vi "status_read.vi"(7 "references":T1, 8 "error in (no error)":errorcluster) -> (0 "error out":errorcluster, 3 "status":T3 {"auto_elapsed_time" format="%<%H:%M:%S%2u>t"})   [LabVIEW 2015, in "lv-recipe-machine.lvlib"]
doc: "This VI can be used to read the current status from the module (public). If you want to ensure that you're getting recently updated data rather than the most recent data, you can include a value for timeout. It's default is 0, in the case the default is used, it returns the most recent value (even if it's never been updated). If the timeout is non-zero and there's no new value, it will output a module specific error noting that the status notifier has timed out."
uses:
  lv-recipe-machine.lvlib
  _controls/status.ctl
  _controls/mode.ctl
  _controls/manual_state.ctl
  _controls/automatic_state.ctl
  _controls/references.ctl
  _controls/input.ctl
  _controls/input_command.ctl
  _controls/output.ctl
  _controls/data.ctl
  _controls/configuration.ctl
  _controls/recipe_data.ctl
  _controls/recipe_step.ctl
  <userlib>/antonio-alexander/lv-waitgroup/public/_controls/api_waitgroup.ctl
  _controls/change.ctl
  <userlib>/antonio-alexander/lv-waitgroup/lv-waitgroup.lvlib
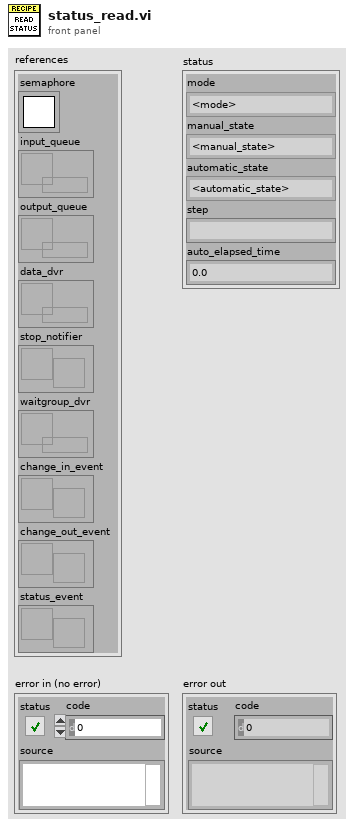
[diagram p1: front panel]
types:
  T1 = typedef "lv-recipe-machine.lvlib/references.ctl" = cluster{"semaphore":T2, "input_queue":refnum<queue>, "output_queue":refnum<queue>, "data_dvr":refnum<data-value>, "stop_notifier":refnum<notifier>, "waitgroup_dvr":refnum<data-value>, "change_in_event":refnum<user-event>, "change_out_event":refnum<user-event>, "status_event":refnum<user-event>}
  T2 = typedef "Semaphore RefNum" = refnum<k1>
  T3 = typedef "lv-recipe-machine.lvlib/status.ctl" = cluster{"mode":T4, "manual_state":T5, "automatic_state":T6, "step":string, "auto_elapsed_time":dbl}
  T4 = typedef "lv-recipe-machine.lvlib/mode.ctl" = enum16{"<mode>", "manual", "automatic", "<null>"}
  T5 = typedef "lv-recipe-machine.lvlib/manual_state.ctl" = enum16{"<manual_state>", "failed", "action", "running", "idle", "<null>"}
  T6 = typedef "lv-recipe-machine.lvlib/automatic_state.ctl" = enum16{"<automatic_state>", "failed", "idle", "running", "paused", "transition", "stopped", "<null>"}
  T7 = typedef "lv-recipe-machine.lvlib/data.ctl" = cluster{"configuration":T8, "working":cluster{"recipe_data":T9, "api_waitgroup":T11}}
  T8 = typedef "lv-recipe-machine.lvlib/configuration.ctl" = cluster{"max_processes":i32}
  T9 = typedef "lv-recipe-machine.lvlib/recipe_data.ctl" = cluster{"mode":T4, "manual_state":T5, "automatic_state":T6, "previous_automatic_state":T6, "error":errorcluster, "manual":cluster{"step_action":string, "data":variant, "actions":variant}, "automatic":cluster{"data":variant, "steps":variant, "criteria":variant, "transition":string, "index":i32, "recipe []":T10[]}}
  T10 = typedef "lv-recipe-machine.lvlib/recipe_step.ctl" = cluster{"step":string, "data":variant}
  T11 = typedef "lv-waitgroup.lvlib/api_waitgroup.ctl" = cluster{"waitgroups":refnum<data-value>, "waitgroup":string}
  T12 = cluster{"step_action":string, "data":variant, "actions":variant}
  T13 = cluster{"data":variant, "steps":variant, "criteria":variant, "transition":string, "index":i32, "recipe []":T10[]}
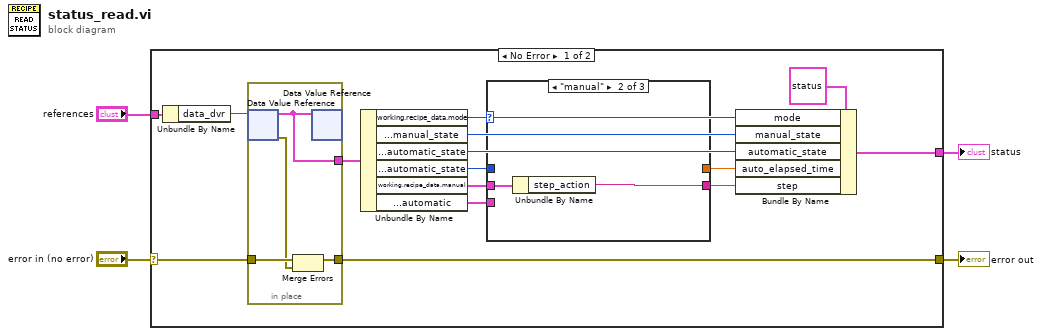
[diagram p0: block diagram]
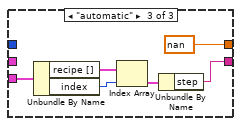
[diagram p3: hidden frame]
diagram:
  n1 = case shown="No Error" "error in (no error)" {
    selector: "error in (no error)" -> [w17 w32]
    tunnel: [w16 w32] -> w3
    tunnel: "references" -> [w19 _]
    tunnel: [w14 _] -> w1
    frame No Error {
      n2 = Unbundle By Name(w19) -> ("data_dvr"=w18:refnum<data-value>)
      n3 = in-place {
        in-place-border: w17 -> [w31]
        in-place-border: [w29] -> w16
        in-place-border: [w28] -> w13
        n4 = in-place-dvr #1(w18) -> (w28:T7, w30:errorcluster)
        n5 = Merge Errors(w31, w30) -> (w29:errorcluster)
        n6 = in-place-dvr #1(w28) -> ()  [unwired: 2 out]
      }
      n7 = Unbundle By Name(w13) -> ("working.recipe_data.mode"=w10:T4, "working.recipe_data.manual_state"=w11:T5, "working.recipe_data.automatic_state"=w12:T6, "working.recipe_data.automatic_state"=w5:T6, "working.recipe_data.manual"=w9:T12, "working.recipe_data.automatic"=w8:T13)
      n8 = case shown="\"manual\"" w10 {
        tunnel: w9 -> [_ w21 _]
        tunnel: w8 -> [_ _ w27]
        tunnel: [_ w20 w23] -> w7
        tunnel: [_ _ nan] -> w6
        tunnel: w5 -> [_ _ _]
        frame Default {
        }
        frame "manual" {
          n9 = Unbundle By Name(w21) -> ("step_action"=w20:string)
        }
        frame "automatic" {
          n10 = Unbundle By Name(w27) -> ("recipe []"=w26:T10[], "index"=w25:i32)
          n11 = Index Array(array=w26, index=w25) -> (element=w24:T10)
          n12 = Unbundle By Name(w24) -> ("step"=w23:string)
        }
      }
      n13 = Bundle By Name(cluster=T3 {"mode"=enum."<mode>", "manual_state"=enum."<manual_state>", "automatic_state"=enum."<automatic_state>", "step"="", "auto_elapsed_time"=0.0} ("status"), "mode"=w10, "manual_state"=w11, "automatic_state"=w12, "auto_elapsed_time"=w6, "step"=w7) -> (w14:T3)
    }
    frame Error {
    }
  }
  "error out" <- w3
  "status" <- w1
